vi "Main_05b raw solution.vi"() -> ()   [LabVIEW 2020]
panel:
  out "concatenated string":string
  out "Array 2":string[](array[string])
  out "Array":string[][](array[string])
  out "Map 2":map{i32, string[]}(c390)
  out "Map":map{i32, string[]}(c390)
  out "array 3":string[](array[string])
  out "array 2":string[](array[string])
  out "sum":i32
  in  "Puzzle":string="[T] [V]                     [W]    \n[V] [C] [P] [D]             [B]    \n[J] [P] [R] [N] [B]         [Z]    \n[W] [Q] [D] [M] [T]     [L] [T]    \n[N] [J] [H] [B] [P] [T] [P] [L]    \n[R] [D] [F] [P] [R] [P] [R] [S] [G]\n[M] [W] [J] [R] [V] [B] [J] [C] [S]\n[S] [B] [B] [F] [H] [C] [B] [N] [L]\n 1   2   3   4   5   6   7   8   9 \n\nmove 7 from 3 to 9\nmove 6 from 2 to 1\nmove 2 from 4 to 8\nmove 10 from 8 to 4\nmove 1 from 2 to 4\nmove 15 from 4 to 1\nmove 28 from 1 to 3\nmove 1 from 2 to 5\nmove 7 from 5 to 9\nmove 5 from 9 to 5\nmove 21 from 3 to 1\nmove 1 from 6 to 4\nmove 4 from 9 to 2\nmove 7 from 9 to 2\nmove 4 from 2 to 6\nmove 1 from 9 to 1\nmove 2 from 4 to 9\nmove 2 from 7 to 4\nmove 4 from 3 to 5\nmove 2 from 7 to 9\nmove 5 from 2 to 7\nmove 2 from 9 to 1\nmove 1 from 9 to 2\nmove 3 from 3 to 7\nmove 3 from 5 to 2\nmove 2 from 6 to 1\nmove 1 from 9 to 4\nmove 25 from 1 to 9\nmove 2 from 5 to 3\nmove 1 from 1 to 7\nmove 9 from 7 to 1\nmove 1 from 2 to 8\nmove 16 from 9 to 7\nmove 5 from 9 to 5\nmove 7 from 1 to 8\nmove 1 from 9 to 7\nmove 18 from 7 to 4\nmove 1 from 3 to 4\nmove 1 from 1 to 8\nmove 2 from 8 to 1\nmove 1 from 3 to 9\nmove 17 from 4 to 5\nmove 5 from 8 to 6\nmove 2 from 8 to 1\nmove 6 from 6 to 7\nmove 2 from 9 to 4\nmove 5 from 1 to 3\nmove 3 from 3 to 7\nmove 1 from 1 to 2\nmove 2 from 3 to 8\nmove 2 from 4 to 1\nmove 2 from 8 to 7\nmove 2 from 9 to 7\nmove 1 from 2 to 4\nmove 1 from 2 to 4\nmove 2 from 1 to 7\nmove 11 from 7 to 1\nmove 4 from 4 to 1\nmove 3 from 1 to 3\nmove 7 from 1 to 8\nmove 4 from 2 to 8\nmove 2 from 1 to 4\nmove 2 from 4 to 3\nmove 2 from 1 to 3\nmove 3 from 7 to 4\nmove 4 from 8 to 6\nmove 1 from 7 to 5\nmove 2 from 4 to 1\nmove 4 from 6 to 2\nmove 3 from 1 to 8\nmove 6 from 8 to 6\nmove 1 from 2 to 1\nmove 23 from 5 to 8\nmove 21 from 8 to 3\nmove 2 from 6 to 9\nmove 1 from 8 to 9\nmove 2 from 3 to 7\nmove 26 from 3 to 8\nmove 2 from 9 to 2\nmove 8 from 6 to 3\nmove 3 from 5 to 4\nmove 1 from 7 to 4\nmove 1 from 7 to 9\nmove 1 from 5 to 4\nmove 5 from 2 to 9\nmove 7 from 9 to 8\nmove 38 from 8 to 7\nmove 1 from 1 to 7\nmove 1 from 4 to 9\nmove 3 from 4 to 1\nmove 4 from 3 to 2\nmove 1 from 1 to 7\nmove 34 from 7 to 6\nmove 3 from 4 to 7\nmove 1 from 4 to 2\nmove 2 from 1 to 3\nmove 1 from 2 to 9\nmove 5 from 3 to 6\nmove 1 from 4 to 6\nmove 4 from 2 to 6\nmove 1 from 9 to 5\nmove 4 from 7 to 3\nmove 1 from 5 to 9\nmove 1 from 9 to 1\nmove 1 from 3 to 6\nmove 1 from 9 to 3\nmove 5 from 7 to 9\nmove 1 from 1 to 9\nmove 3 from 9 to 1\nmove 1 from 3 to 4\nmove 38 from 6 to 1\nmove 2 from 9 to 4\nmove 3 from 3 to 6\nmove 1 from 9 to 5\nmove 8 from 6 to 8\nmove 1 from 3 to 6\nmove 1 from 6 to 8\nmove 2 from 4 to 3\nmove 4 from 8 to 5\nmove 1 from 6 to 2\nmove 1 from 2 to 7\nmove 1 from 6 to 3\nmove 3 from 8 to 7\nmove 4 from 7 to 6\nmove 1 from 4 to 1\nmove 5 from 1 to 4\nmove 4 from 6 to 5\nmove 3 from 5 to 8\nmove 3 from 5 to 3\nmove 1 from 8 to 2\nmove 6 from 3 to 8\nmove 1 from 5 to 7\nmove 1 from 2 to 1\nmove 1 from 7 to 6\nmove 3 from 4 to 9\nmove 6 from 8 to 6\nmove 3 from 8 to 2\nmove 3 from 6 to 2\nmove 1 from 4 to 5\nmove 1 from 6 to 9\nmove 2 from 6 to 1\nmove 1 from 4 to 1\nmove 2 from 5 to 2\nmove 1 from 8 to 5\nmove 1 from 9 to 8\nmove 22 from 1 to 5\nmove 3 from 2 to 3\nmove 1 from 8 to 4\nmove 2 from 3 to 6\nmove 1 from 6 to 4\nmove 1 from 3 to 8\nmove 1 from 2 to 8\nmove 10 from 5 to 3\nmove 1 from 6 to 8\nmove 2 from 8 to 4\nmove 1 from 6 to 3\nmove 2 from 2 to 3\nmove 1 from 8 to 5\nmove 13 from 3 to 4\nmove 2 from 1 to 7\nmove 11 from 1 to 2\nmove 3 from 4 to 5\nmove 6 from 1 to 9\nmove 8 from 2 to 6\nmove 4 from 2 to 1\nmove 2 from 6 to 5\nmove 4 from 1 to 8\nmove 2 from 8 to 6\nmove 1 from 7 to 1\nmove 1 from 7 to 2\nmove 8 from 6 to 5\nmove 1 from 8 to 4\nmove 1 from 1 to 6\nmove 10 from 5 to 1\nmove 3 from 9 to 4\nmove 6 from 1 to 3\nmove 9 from 4 to 5\nmove 1 from 2 to 1\nmove 1 from 4 to 9\nmove 1 from 6 to 8\nmove 1 from 2 to 1\nmove 1 from 4 to 8\nmove 2 from 8 to 9\nmove 1 from 8 to 6\nmove 1 from 3 to 2\nmove 1 from 1 to 4\nmove 1 from 2 to 5\nmove 1 from 1 to 8\nmove 1 from 6 to 8\nmove 8 from 5 to 3\nmove 1 from 8 to 7\nmove 1 from 7 to 8\nmove 6 from 9 to 6\nmove 2 from 9 to 2\nmove 1 from 9 to 7\nmove 1 from 8 to 5\nmove 1 from 2 to 7\nmove 1 from 2 to 9\nmove 16 from 5 to 2\nmove 4 from 5 to 1\nmove 12 from 3 to 6\nmove 1 from 5 to 4\nmove 8 from 6 to 9\nmove 1 from 8 to 5\nmove 2 from 9 to 6\nmove 2 from 2 to 5\nmove 3 from 1 to 4\nmove 3 from 6 to 7\nmove 7 from 9 to 6\nmove 4 from 7 to 1\nmove 1 from 5 to 2\nmove 1 from 3 to 2\nmove 4 from 1 to 9\nmove 4 from 9 to 5\nmove 12 from 6 to 7\nmove 4 from 2 to 6\nmove 4 from 2 to 9\nmove 7 from 6 to 3\nmove 3 from 9 to 8\nmove 5 from 2 to 4\nmove 4 from 5 to 7\nmove 1 from 9 to 4\nmove 13 from 7 to 8\nmove 3 from 7 to 8\nmove 2 from 3 to 2\nmove 5 from 1 to 5\nmove 11 from 4 to 9\nmove 7 from 9 to 1\nmove 4 from 4 to 3\nmove 1 from 6 to 8\nmove 8 from 8 to 4\nmove 1 from 1 to 7\nmove 3 from 4 to 6\nmove 4 from 2 to 8\nmove 3 from 5 to 4\nmove 1 from 4 to 1\nmove 4 from 9 to 8\nmove 3 from 5 to 2\nmove 2 from 2 to 3\nmove 1 from 6 to 7\nmove 7 from 1 to 9\nmove 3 from 7 to 4\nmove 1 from 4 to 2\nmove 1 from 6 to 8\nmove 1 from 5 to 7\nmove 1 from 6 to 7\nmove 9 from 4 to 6\nmove 7 from 9 to 5\nmove 1 from 4 to 3\nmove 1 from 5 to 6\nmove 4 from 3 to 7\nmove 3 from 3 to 1\nmove 2 from 2 to 4\nmove 3 from 1 to 6\nmove 4 from 5 to 1\nmove 2 from 5 to 3\nmove 3 from 6 to 8\nmove 6 from 7 to 3\nmove 10 from 3 to 7\nmove 10 from 6 to 4\nmove 3 from 1 to 9\nmove 4 from 7 to 2\nmove 2 from 3 to 5\nmove 1 from 3 to 5\nmove 1 from 1 to 2\nmove 3 from 9 to 1\nmove 2 from 1 to 9\nmove 4 from 2 to 5\nmove 10 from 4 to 9\nmove 2 from 8 to 7\nmove 1 from 2 to 9\nmove 1 from 9 to 4\nmove 1 from 1 to 9\nmove 3 from 7 to 8\nmove 5 from 9 to 8\nmove 6 from 5 to 4\nmove 5 from 9 to 6\nmove 5 from 8 to 5\nmove 4 from 5 to 2\nmove 3 from 7 to 8\nmove 3 from 9 to 1\nmove 2 from 5 to 8\nmove 1 from 4 to 6\nmove 3 from 6 to 3\nmove 8 from 4 to 3\nmove 2 from 6 to 7\nmove 24 from 8 to 9\nmove 1 from 6 to 9\nmove 8 from 9 to 3\nmove 1 from 1 to 9\nmove 2 from 8 to 3\nmove 3 from 9 to 4\nmove 18 from 3 to 5\nmove 1 from 2 to 6\nmove 1 from 6 to 1\nmove 13 from 9 to 8\nmove 3 from 4 to 1\nmove 1 from 4 to 2\nmove 1 from 5 to 3\nmove 1 from 9 to 2\nmove 6 from 2 to 9\nmove 3 from 3 to 1\nmove 3 from 7 to 6\nmove 2 from 1 to 5\nmove 3 from 6 to 7\nmove 17 from 8 to 1\nmove 8 from 5 to 7\nmove 11 from 7 to 5\nmove 1 from 4 to 5\nmove 24 from 1 to 3\nmove 7 from 5 to 9\nmove 11 from 5 to 9\nmove 1 from 5 to 4\nmove 1 from 5 to 2\nmove 1 from 4 to 7\nmove 16 from 3 to 1\nmove 3 from 5 to 8\nmove 1 from 9 to 1\nmove 12 from 9 to 2\nmove 5 from 3 to 1\nmove 2 from 8 to 5\nmove 2 from 3 to 4\nmove 1 from 8 to 6\nmove 2 from 5 to 3\nmove 1 from 6 to 1\nmove 2 from 4 to 1\nmove 8 from 2 to 1\nmove 24 from 1 to 6\nmove 1 from 9 to 6\nmove 4 from 2 to 6\nmove 4 from 3 to 2\nmove 4 from 9 to 4\nmove 1 from 7 to 5\nmove 6 from 9 to 1\nmove 17 from 6 to 4\nmove 1 from 1 to 9\nmove 2 from 9 to 7\nmove 9 from 6 to 7\nmove 12 from 7 to 2\nmove 11 from 1 to 2\nmove 12 from 4 to 2\nmove 1 from 1 to 4\nmove 1 from 5 to 7\nmove 2 from 6 to 3\nmove 2 from 4 to 3\nmove 1 from 1 to 6\nmove 5 from 4 to 2\nmove 1 from 7 to 5\nmove 2 from 6 to 9\nmove 6 from 2 to 4\nmove 1 from 5 to 8\nmove 3 from 4 to 1\nmove 1 from 8 to 9\nmove 5 from 4 to 1\nmove 1 from 1 to 2\nmove 1 from 3 to 8\nmove 7 from 1 to 6\nmove 1 from 8 to 6\nmove 1 from 3 to 5\nmove 1 from 1 to 8\nmove 1 from 4 to 5\nmove 2 from 5 to 9\nmove 1 from 8 to 2\nmove 2 from 6 to 8\nmove 1 from 8 to 6\nmove 1 from 6 to 8\nmove 1 from 8 to 5\nmove 4 from 9 to 5\nmove 1 from 9 to 6\nmove 1 from 6 to 8\nmove 37 from 2 to 5\nmove 1 from 2 to 8\nmove 37 from 5 to 8\nmove 21 from 8 to 4\nmove 1 from 3 to 7\nmove 12 from 4 to 1\nmove 1 from 7 to 8\nmove 4 from 6 to 3\nmove 1 from 4 to 2\nmove 2 from 2 to 6\nmove 2 from 3 to 2\nmove 2 from 2 to 7\nmove 2 from 7 to 1\nmove 3 from 5 to 3\nmove 2 from 2 to 8\nmove 15 from 8 to 7\nmove 1 from 7 to 2\nmove 2 from 5 to 8\nmove 5 from 4 to 3\nmove 3 from 6 to 2\nmove 8 from 1 to 9\nmove 8 from 9 to 4\nmove 7 from 8 to 9\nmove 2 from 8 to 5\nmove 4 from 1 to 9\nmove 10 from 3 to 2\nmove 1 from 6 to 7\nmove 6 from 7 to 8\nmove 10 from 4 to 7\nmove 1 from 3 to 7\nmove 3 from 9 to 1\nmove 5 from 8 to 1\nmove 5 from 2 to 7\nmove 1 from 4 to 3\nmove 1 from 5 to 6\nmove 10 from 1 to 7\nmove 34 from 7 to 4\nmove 1 from 6 to 9\nmove 1 from 7 to 3\nmove 8 from 4 to 2\nmove 1 from 9 to 7\nmove 1 from 7 to 9\nmove 22 from 4 to 5\nmove 1 from 3 to 8\nmove 6 from 5 to 6\nmove 1 from 8 to 4\nmove 9 from 9 to 4\nmove 1 from 3 to 2\nmove 4 from 2 to 1\nmove 11 from 2 to 6\nmove 14 from 4 to 7\nmove 1 from 2 to 1\nmove 12 from 5 to 6\nmove 7 from 7 to 9\nmove 2 from 5 to 4\nmove 1 from 8 to 5\nmove 6 from 6 to 8\nmove 3 from 7 to 8\nmove 1 from 2 to 6\nmove 2 from 4 to 3\nmove 1 from 3 to 8\nmove 1 from 2 to 5\nmove 1 from 3 to 4\nmove 5 from 8 to 9\nmove 5 from 1 to 4\nmove 3 from 8 to 9\nmove 5 from 4 to 7\nmove 18 from 6 to 3\nmove 2 from 8 to 9\nmove 3 from 6 to 3\nmove 5 from 7 to 1\nmove 1 from 6 to 7\nmove 3 from 9 to 7\nmove 6 from 7 to 8\nmove 8 from 9 to 8\nmove 1 from 7 to 6\nmove 12 from 3 to 1\nmove 2 from 9 to 7\nmove 1 from 8 to 6\nmove 9 from 8 to 9\nmove 2 from 8 to 7\nmove 1 from 7 to 8\nmove 2 from 1 to 6\nmove 7 from 1 to 9\nmove 16 from 9 to 5\nmove 4 from 3 to 9\nmove 8 from 1 to 3\nmove 5 from 5 to 1\nmove 1 from 4 to 3\nmove 4 from 7 to 6\nmove 3 from 8 to 2\nmove 8 from 3 to 2\nmove 11 from 2 to 7\nmove 3 from 6 to 1\nmove 4 from 3 to 6\nmove 12 from 5 to 7\nmove 2 from 3 to 6\nmove 7 from 1 to 7\nmove 2 from 5 to 1\nmove 1 from 9 to 2\nmove 1 from 5 to 7\nmove 31 from 7 to 4\nmove 6 from 9 to 1\nmove 6 from 4 to 7\nmove 16 from 4 to 5\nmove 1 from 9 to 4\nmove 1 from 7 to 6\nmove 4 from 4 to 1\nmove 11 from 5 to 9\nmove 2 from 5 to 6\nmove 1 from 2 to 9\nmove 4 from 5 to 1\nmove 8 from 9 to 2\nmove 12 from 6 to 5\nmove 11 from 5 to 1\nmove 18 from 1 to 2\nmove 3 from 4 to 3\nmove 2 from 6 to 7\nmove 2 from 9 to 1\nmove 1 from 5 to 9\nmove 3 from 9 to 5\nmove 13 from 2 to 8\nmove 10 from 8 to 2\nmove 3 from 8 to 6\nmove 3 from 3 to 9\nmove 7 from 1 to 5\nmove 6 from 5 to 6\nmove 3 from 1 to 2\nmove 5 from 7 to 8\nmove 13 from 2 to 8\nmove 9 from 6 to 3"
  in  "Example":string="    [D]    \n[N] [C]    \n[Z] [M] [P]\n 1   2   3 \n\nmove 1 from 2 to 1\nmove 3 from 1 to 3\nmove 2 from 2 to 1\nmove 1 from 1 to 2"
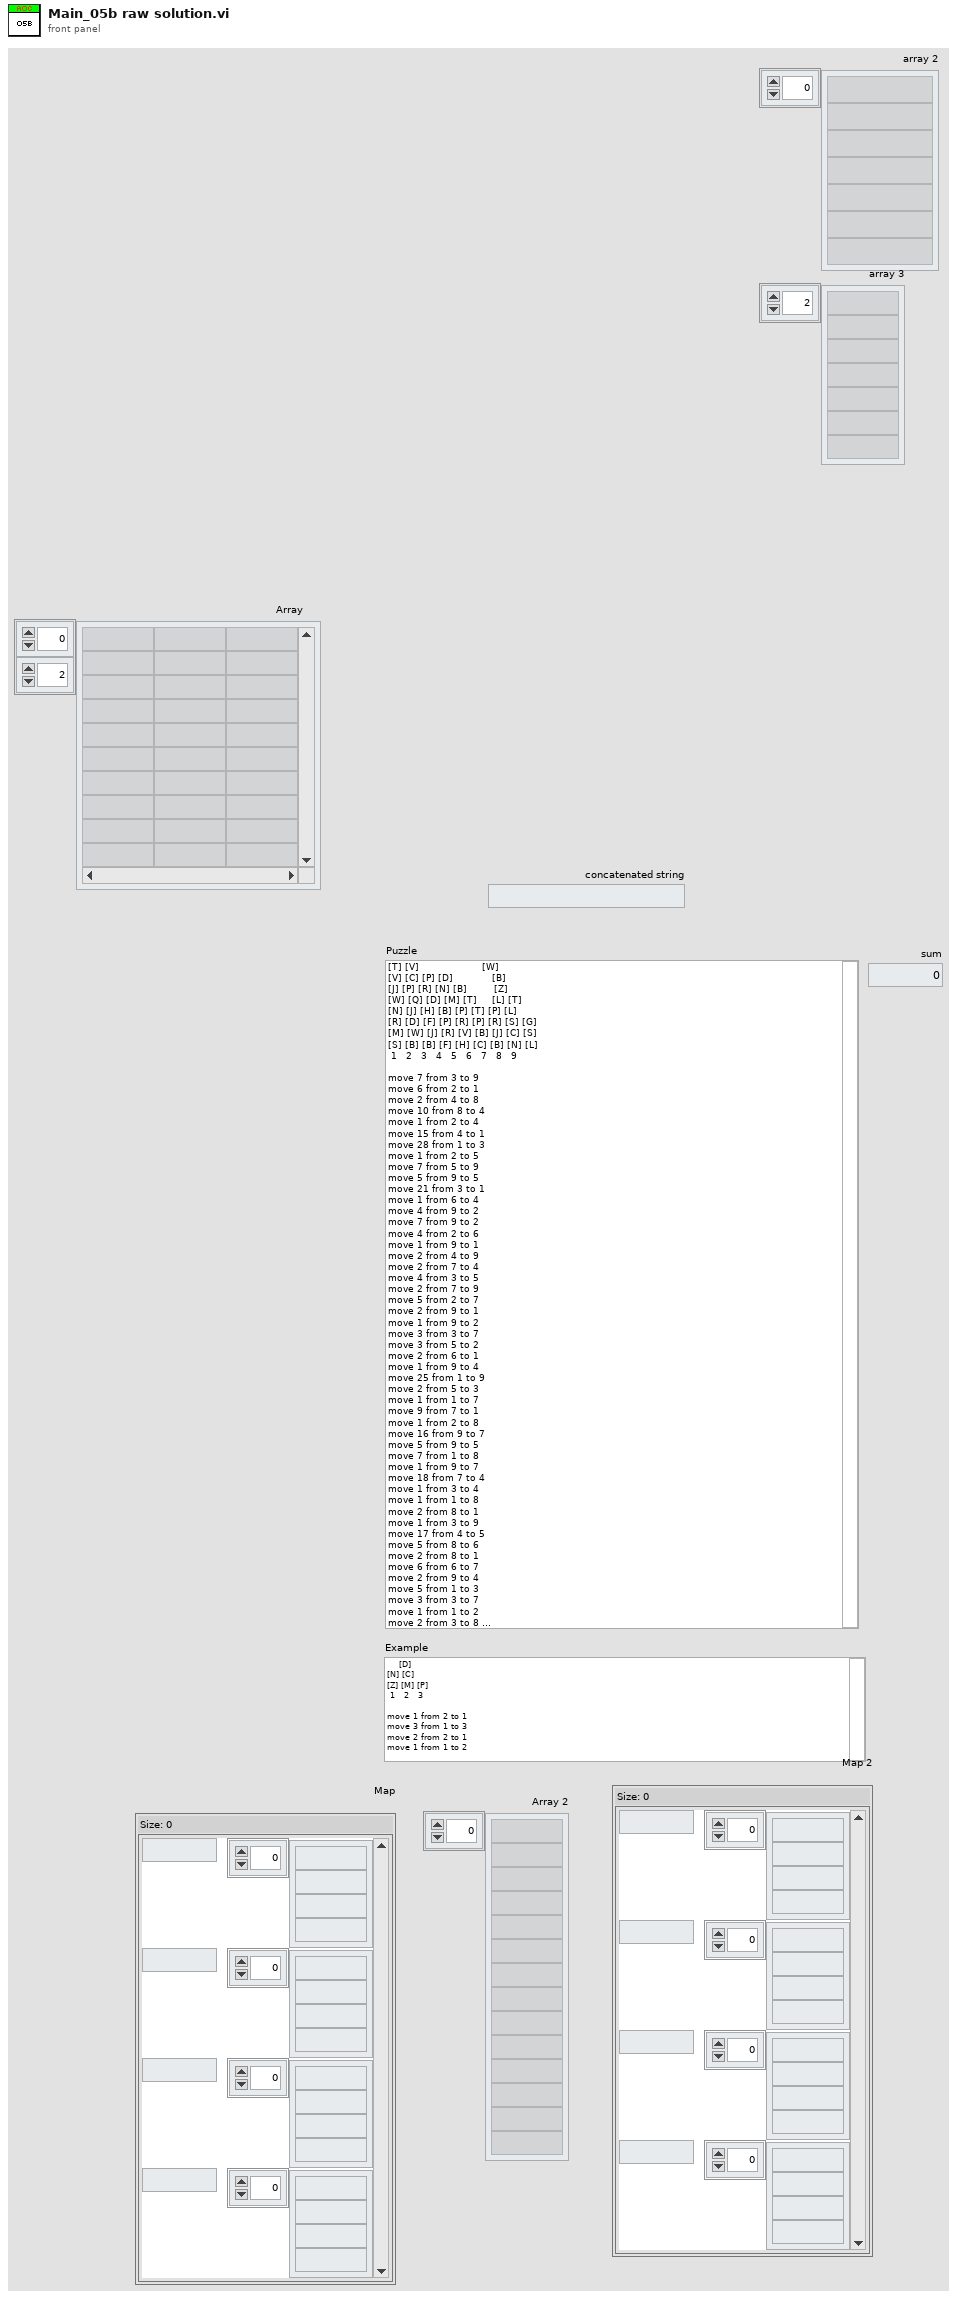
[diagram p1: front panel]
types:
  T1 = cluster{"Count":i32, "Start Pile":i32, "End Pile":i32}
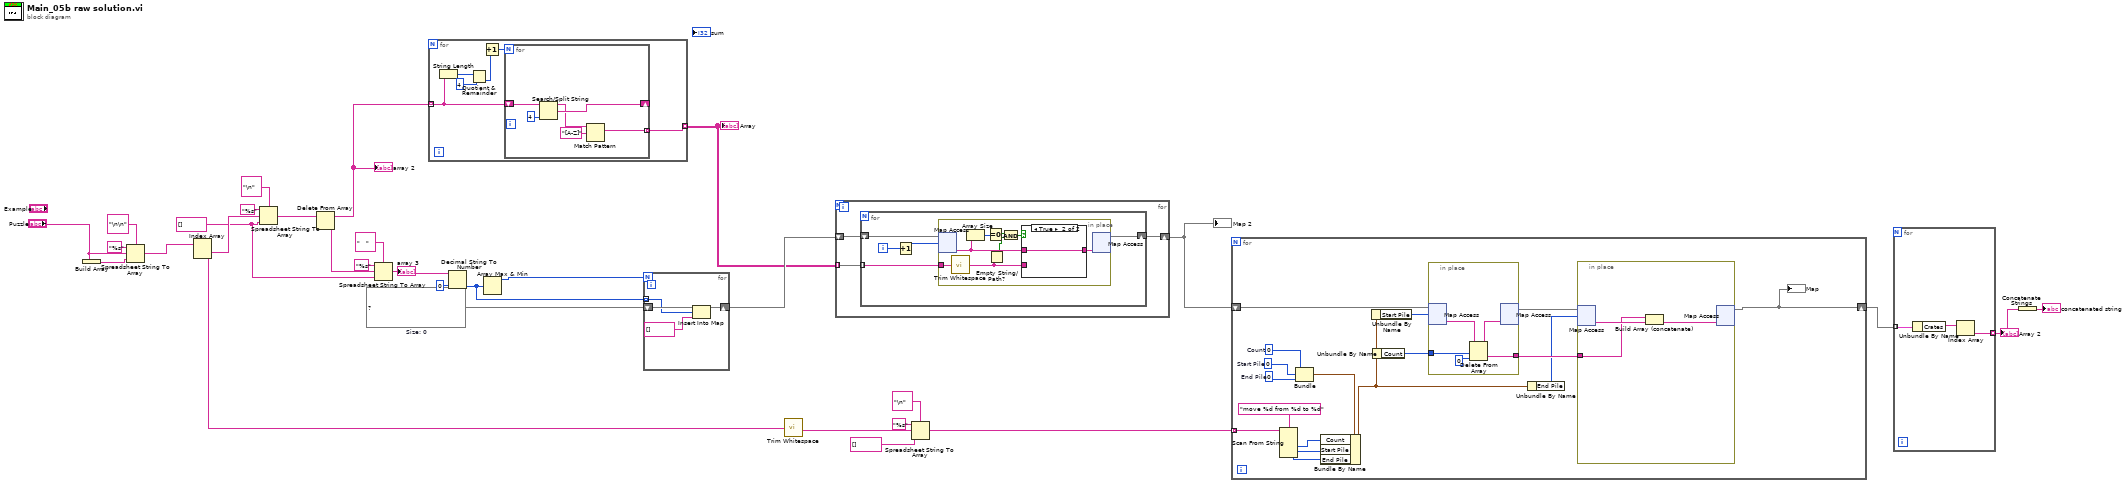
[diagram p0: block diagram]
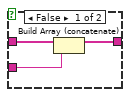
[diagram p2: hidden frame]
diagram:
  w16 = map{i32, string[]} {}  # Size: 0
  w20 = string[] [] ("appended array")
  n1 = Build Array("Puzzle") -> (w31:string[])
  n2 = Spreadsheet String To Array(delimiter (Tab)="\n\n", format string="%s", spreadsheet string="Puzzle", array type (2D Dbl)=w31) -> (array=w28:string[])
  n3 = Index Array(array=w28) -> (element #1=w25:string, element #2=w13:string)  [unwired: 2 in]
  n4 = Spreadsheet String To Array(delimiter (Tab)="\n", format string="%s", spreadsheet string=w25, array type (2D Dbl)=w20) -> (array=w24:string[])
  n5 = Delete From Array(array=w24) -> (deleted portion=w21:string, array with subset deleted=w6:string[])  [unwired: 2 in]
  "array 2" <- w6
  n6 = Spreadsheet String To Array(delimiter (Tab)="   ", format string="%s", spreadsheet string=w21, array type (2D Dbl)=w20) -> (array=w19:string[])
  "array 3" <- w19
  n7 = for {
    tunnel: w6 -> [w34] mode=indexing
    tunnel: [w33] -> w5 mode=indexing
    n8 = String Length(string=w34) -> (length=w37:i32)
    n9 = Quotient & Remainder(x=w37, y=4) -> (floor(x/y)=w35:i32)  [unwired: 1 out]
    n10 = Increment(x=w35) -> (x+1=w32:i32)
    n11 = for {
      N: w32 -> [_]
      shift-right: [w42] -> _
      shift-left: w34 -> [w43]
      tunnel: [w38] -> w33 mode=indexing
      n12 = Search/Split String(string=w43, offset (0)=4) -> (substring before match=w40:string, match + rest of string=w42:string)  [unwired: 1 in, 1 out]
      n13 = Match Pattern(string=w40, regular expression="[A-Z]") -> (match substring=w38:string)  [unwired: 1 in, 3 out]
    }
  }
  "Array" <- w5
  n14 = Decimal String To Number(string=w19, default (0L)=0 ("default (0 I32)")) -> (number=w15:i32[])  [unwired: 1 in, 1 out]
  n15 = Array Max & Min(array=w15) -> (max value=w17:i32)  [unwired: 3 out]
  n16 = for {
    N: w17 -> [_]
    shift-right: [w46] -> w14
    shift-left: w16 -> [w47]
    tunnel: w15 -> [w44] mode=indexing
    n17 = Insert Into Map(map in=w47, key=w44, value=string[] []) -> (map out=w46:map{i32, string[]})  [unwired: 2 out]
  }
  n18 = call <vilib>:"Trim Whitespace.vi"("string"=w13) -> ("trimmed string"=w10:string)  [unwired: 1 in]
  n19 = for {
    shift-right: [w48] -> w7
    shift-left: w14 -> [w50]
    tunnel: w5 -> [w49] mode=indexing
    n20 = for {
      shift-right: [w52] -> w48
      shift-left: w50 -> [w55]
      tunnel: w49 -> [w51] mode=indexing
      i -> [w54]
      n21 = Increment(x=w54) -> (x+1=w53:i32)
      n22 = in-place {
        in-place-border: w51 -> [w60]
        n23 = in-place-map #1(w55, w53) -> (w62:string[])  [unwired: 1 in, 1 out]
        n24 = call <vilib>:"Trim Whitespace.vi"("string"=w60) -> ("trimmed string"=w59:string)  [unwired: 1 in]
        n25 = Array Size(array=w62) -> (size(s)=w61:i32)
        n26 = Equal To 0?(x=w61) -> (x = 0?=w57:bool)
        n27 = Empty String/Path?(string/path=w59) -> (empty?=w58:bool)
        n28 = And(x=w57, y=w58) -> (x .and. y?=w56:bool)
        n29 = case shown="True" w56 {
          tunnel: [w66 w67] -> w63
          tunnel: w59 -> [w65 _]
          tunnel: w62 -> [w64 w67]
          frame False {
            n30 = Build Array (concatenate)(w64, w65) -> (w66:string[])
          }
          frame True {
          }
        }
        n31 = in-place-map #1(w63) -> (w52:map{i32, string[]})  [unwired: 1 in, 2 out]
      }
    }
  }
  "Map 2" <- w7
  n32 = Spreadsheet String To Array(delimiter (Tab)="\n", format string="%s", spreadsheet string=w10, array type (2D Dbl)=string[] [] ("value")) -> (array=w8:string[])
  n33 = for {
    tunnel: w8 -> [w76] mode=indexing
    shift-right: [w72] -> w4
    shift-left: w7 -> [w75]
    w84 = 0  # End Pile
    w80 = 0  # Count
    w83 = 0  # Start Pile
    n34 = Scan From String(format string="move %d from %d to %d", input string=w76) -> (output 1=w78:i32, output 2=w79:i32, output 3=w77:i32)  [unwired: 5 in, 3 out]
    n35 = Bundle("Count"=w80, "Start Pile"=w83, "End Pile"=w84) -> (w81:T1)  [unwired: 1 in]
    n36 = Bundle By Name(cluster=w81, "Count"=w78, "Start Pile"=w79, "End Pile"=w77) -> (w73:T1)
    n37 = Unbundle By Name(w73) -> ("Start Pile"=w74:i32)
    n38 = Unbundle By Name(w73) -> ("Count"=w68:i32)
    n39 = in-place {
      in-place-border: [w89] -> w70
      in-place-border: w68 -> [w88]
      n40 = in-place-map #2(w75, w74) -> (w92:string[])  [unwired: 1 in, 1 out]
      n41 = Delete From Array(array=w92, length=w88, index=0) -> (deleted portion=w89:string[], array with subset deleted=w91:string[])
      n42 = in-place-map #2(w91) -> (w71:map{i32, string[]})  [unwired: 1 in, 2 out]
    }
    n43 = Unbundle By Name(w73) -> ("End Pile"=w69:i32)
    n44 = in-place {
      in-place-border: w70 -> [w85]
      n45 = in-place-map #3(w71, w69) -> (w87:string[])  [unwired: 1 in, 1 out]
      n46 = Build Array (concatenate)(w85, w87) -> (w86:string[])
      n47 = in-place-map #3(w86) -> (w72:map{i32, string[]})  [unwired: 1 in, 2 out]
    }
    "Map" <- w72
  }
  n48 = for {
    tunnel: w4 -> [w95] mode=indexing
    tunnel: [w93] -> w3 mode=indexing
    n49 = Unbundle By Name(w95) -> ("Crates"=w94:string[])
    n50 = Index Array(array=w94) -> (element=w93:string)  [unwired: 1 in]
  }
  "Array 2" <- w3
  n51 = Concatenate Strings(w3) -> (→"concatenated string":string)
